vi "Rx Streaming Time (Host).vi"() -> ()   [LabVIEW 2021]
doc: "This template is for the Simple NI-USRP Streaming design, a design that shows the basics of streaming data to and from an NI USRP-294x/295x device. Refer to the block diagram for more information about how to use this template."
uses:
  Host/SubVIs/Start Trigger.ctl
  <extravilib>/ChannelInstances/Tag-c(bool,i32,str).lvlib
  <extravilib>/ChannelInstances/Stream-u32.lvlib
  <extravilib>/ChannelInstances/Tag-bool.lvlib
  <vilib>/userDefined/Silver/nirio_resource_slv.ctl
panel:
  out "acquiring":bool caption="Streaming"
  out "write time":u32[](graph)
  in  "max queue size":i32=100
  out "record time (ms)":u32
  out "write rate (SPS)":dbl format="%#_6p"
  out "# elements in queue":i32
  out "write tdms loop time (ms)":u32
  in  "frequency":dbl=2000000000.0 format="%#_6p"
  in  "sample rate":i32=50000000 format="%.0p"
  in  "start trigger":T1=enum."Immediate"
  out "get data loop time (ms)":u32 format="%.0p"
  out "error tdms_loop":errorcluster
  in  "USRP RIO device":T2="RIO0" caption="USRP RIO Device"
  in  "rx.stop":bool
  # "Overview: Demonstrates the use of the Advanced TDMS and simple streamer functions to write Rx data to a *.tdms file.\nInstructions:\nThis Vi must use Administrator privliges in order to write the data.\nthe USRP sohld be connected via MIXe to the computer (or other direct connection)\nset the params \nRun this VI.\ndue to the way the memory work after some time it can occer that the saveing rate will decrise."
  # "Rx Streaming"
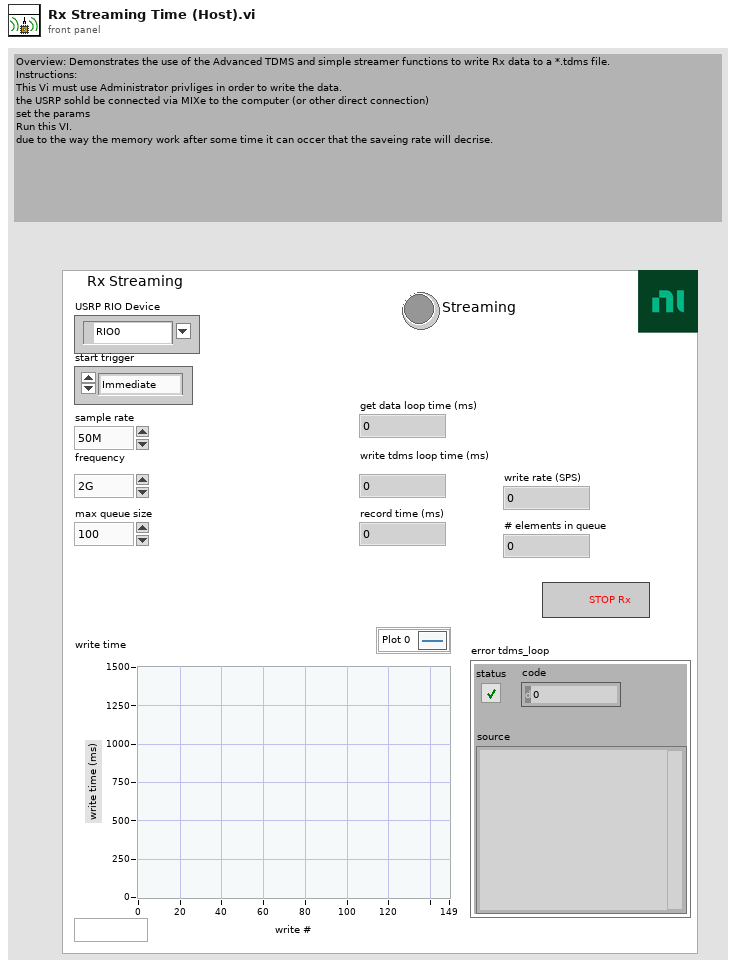
[diagram p1: front panel]
types:
  T1 = typedef "Start Trigger.ctl" = enum8{"Software", "Digital Edge", "Rx Start Trigger", "Tx Start Trigger", "Immediate", "Future Time Event"}
  T2 = typedef "nirio_resource_slv.ctl" = tag
  T3 = cluster{"rf enable 0":bool, "rf config 0":cluster{"antenna":string, "frequency":dbl, "lo frequency":dbl, "level":dbl}, "rf enable 1":bool, "rf config 1":cluster{"antenna":string, "frequency":dbl, "lo frequency":dbl, "level":dbl}, "transfer mode":enum16{"Finite", "Continuous"}, "sample rate":dbl, "number of samples":u32, "start trigger":T1}
  T4 = enum16{"open", "open or create", "create or replace", "create", "open (read-only)"}
  T5 = typedef "Rx Channels.ctl" = cluster{"rx config":cluster{"channel configuration":cluster{"channel enable":bool, "channel configuration":cluster{"antenna":string, "frequency":dbl, "lo frequency":dbl, "level":dbl}}[], "transfer mode":enum16{"Finite", "Continuous"}, "sample rate":dbl, "number of samples":u32, "start trigger":T1}, "reference frequency source":string, "rx.data sink":enum16{"SFP Port 0", "SFP Port 1", "Host"}, "rx.enabled channels":string[], "vertical range":dbl[], "rx.coerced configurations":cluster{"coerced frequencies":dbl[], "coerced lo frequencies":dbl[], "coerced levels":dbl[], "coerced sample rates":dbl[]}}
  T6 = typedef "niUsrpRio Config v1 Host.lvlib/niUsrpRio Session.ctl" = cluster{"FPGA Interface":refnum<k20>, "RIO Interface Number":u32, "Data Clock Rate":u32, "FPGA Data Clock Rate":u32, "Global Settings Register Bus":T7, "Radio 0 Settings Register Bus":T7, "Radio 1 Settings Register Bus":T7, "Radio Settings Bus Semaphore":T8, "DB Queues":T9[], "Characterization Data Valid?":bool, "EEPROM Header":T10, "Device Data Header":T11, "EEPROM Characterization Header":T12, "Characterization Data":T13[], "FPGA Current Version":u32, "FPGA Oldest Compatible Version":u32, "Fixed Logic Current Version":u32, "Fixed Logic Oldest Compatible Version":u32, "FPGA Radio Settings Bus Current Version":u32, "FPGA Radio Settings Bus Oldest Compatible Version":u32, "FPGA Board Config Current Version":u32, "FPGA Board Config Oldest Compatible Version":u32, "Daughterboard Clock Rate":u32, "daughterboard configuration session handles":u64[]}
  T7 = typedef "niInstr Register Bus v0 Host.lvlib/Register Bus Session.ctl" = refnum<queue>
  T8 = typedef "Semaphore RefNum" = refnum<k1>
  T9 = typedef "niUsrpRio Config v1 Host.lvlib/DB Queue Reference.ctl" = refnum<queue>
  T10 = typedef "niUsrpRio Config v1 Host.lvlib/EEPROM Header.ctl" = cluster{"Checksum":u32, "Product Code":u16, "Hardware Current Version":u16, "Hardware Oldest Compatible Version":u16, "EEPROM Map Current Version":u16, "EEPROM Map Oldest Compatible Version":u16, "User Password":string, "Pointer to Factory Header":u32, "Pointer to User Header":u32, "Recommended Interval":u16, "Number of Reserved Bytes":i32, "Number of Daughterboards":u8, "Daughterboard IDs":u16[], "Daughterboard Serial Numbers":string[]}
  T11 = typedef "niUsrpRio Config v1 Host.lvlib/EEPROM Device Data Header.ctl" = cluster{"Checksum":u32, "Number of Channels":u8, "Number of Gain Settings":u16[], "Pointer to Characterization Data":u32[], "Number of Reserved Bytes":i32, "Number of Frequencies":u16[]}
  T12 = typedef "niUsrpRio Config v1 Host.lvlib/EEPROM Characterization Header.ctl" = cluster{"Checksum":u32, "Date":timestamp, "Temperature":sgl, "Misc. Info":string, "Pointer to Device Data Header":u32, "Number of Reserved Bytes":i32}
  T13 = typedef "niUsrpRio Config v1 Host.lvlib/Characterization Data.ctl" = cluster{"Gains[dB]":dbl[], "Frequencies [Hz]":dbl[], "IQ Imbalance Table":T14[], "Measured Gains[dB]":dbl[][]}
  T14 = typedef "niUsrpRio Config v1 Host.lvlib/IQ Imbalance.ctl" = cluster{"Gain Imbalance [linear]":dbl, "Phase Imbalance [radians]":dbl, "Offset":cdb}
  T15 = typedef "Tag-bool.lvlib/))Channel.ctl" = refnum<queue>
  T16 = typedef "Stream-u32.lvlib/)Channel.ctl" = refnum<queue>
  T17 = typedef "Tag-c(bool,i32,str).lvlib/))Channel.ctl" = refnum<queue>
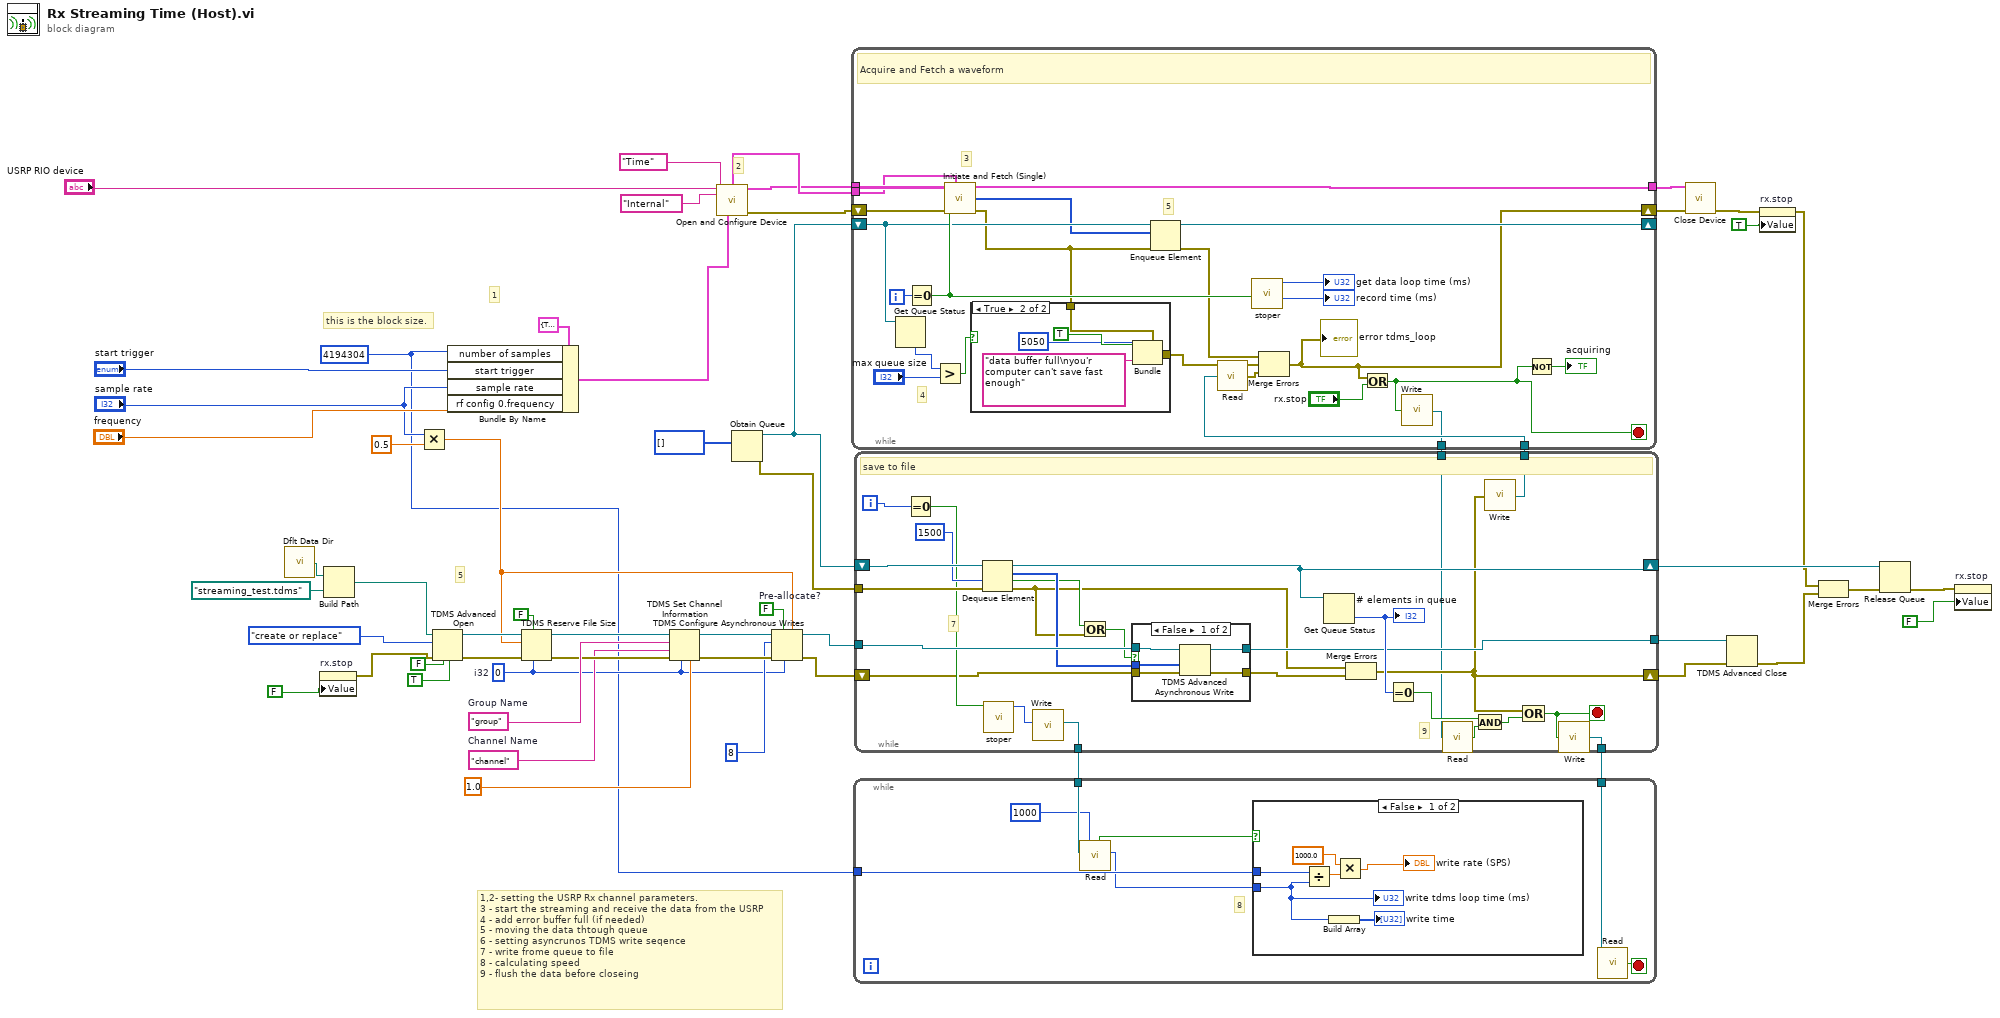
[diagram p0: block diagram]
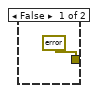
[diagram p3: hidden frame]
diagram:
  w5 = 4194304
  w43 = FALSE  # Pre-allocate?
  w21 = 0  # i32
  w54 = "group"  # Group Name
  w23 = "channel"  # Channel Name
  # "1,2- setting the USRP Rx channel parameters.\n3 - start the streaming and receive the data from the USRP\n4 - add error buffer full (if needed)\n5 - moving the data thtough queue   \n6 - setting asyncrunos TDMS write seqence\n7 - write frome queue to file\n8 - calculating speed\n9 - flush the data before closeing"
  # "5"
  # "2"
  # "1"
  # "this is the block size."
  n1 = call <vilib>:"Dflt Data Dir.vi"() -> ("App:Default Data Directory"=w10:path)
  n2 = property on="rx.stop" class="Bool (strict)"("Value"=FALSE) -> (error out=w16:errorcluster)  [unwired: 2 in, 1 out]
  n3 = Build Path(base path=w10, name or relative path=path "streaming_test.tdms") -> (appended path=w9:path)
  n4 = Multiply(x="sample rate", y=0.5) -> (x*y=w24:dbl)
  n5 = TDMS Advanced Open(4:TRUE ("enable asynchronous? (T)"), 6:FALSE ("disable buffering? (T)"), 8:w16, 10:T4."create or replace" ("operation (0:open)"), 11:w9) -> (0:w50:errorcluster, 3:w51:refnum<k34>)  [unwired: 1 out]
  n6 = Bundle By Name(cluster=T3 {"rf enable 0"=TRUE, "rf config 0"={"antenna"="RX1", "frequency"=2000000000.0, "lo frequency"=-1.0, "level"=0.0}, "rf enable 1"=FALSE, "rf config 1"={"antenna"="RX2", "frequency"=2000000000.0, "lo frequency"=-1.0, "level"=0.0}, "transfer mode"=enum."Continuous", "sample rate"=10000000.0, "number of samples"=4194304, "start trigger"=enum."Immediate"} ("rx config"), "number of samples"=w5, "start trigger"="start trigger", "sample rate"="sample rate", "rf config 0.frequency"="frequency") -> (w46:T3)
  n7 = TDMS Reserve File Size(6:w21, 7:FALSE ("append? (T)"), 8:w50, 10:w24, 11:w51) -> (0:w48:errorcluster, 3:w49:refnum<k34>)
  n8 = TDMS Set Channel Information(4:1.0 ("y"), 6:w21, 8:w48, 9:w23, 10:w54, 11:w49) -> (0:w45:errorcluster, 3:w44:refnum<k34>)  [unwired: 1 in]
  n9 = call "Open and Configure Device.vi"("USRP RIO Device"="USRP RIO device", "reference frequency source"="Internal", "which bitfile"="Time", "rx config"=w46) -> ("rx channels"=w56:T5, "niUsrpRio Session (out)"=w42:T6, "error out"=w41:errorcluster)  [unwired: 5 in, 4 out]
  n10 = Obtain Queue(element data type=u32[] [] ("waveform data")) -> (queue out=w30:refnum<queue>, error out=w29:errorcluster)  [unwired: 4 in, 1 out]
  n11 = TDMS Configure Asynchronous Writes(5:w24, 6:w21, 7:w43, 8:w45, 10:u32 8 ("max asynchronous writes (4)"), 11:w44) -> (0:w25:errorcluster, 3:w31:refnum<k34>)  [unwired: 1 in]
  n12 = while {
    tunnel: w42 -> [w78]
    tunnel: [w75] -> w32
    tunnel: w56 -> [w76]
    shift-right: [w74] -> _
    shift-left: w30 -> [w71]
    tunnel: w6 -> [w61]
    tunnel: [w60] -> w1
    shift-right: [w57] -> w8
    shift-left: w41 -> [w79]
    i -> [w80]
    stop <- w59 stop-if-true
    # "5"
    # "4"
    # "3"
    # "Acquire and Fetch a waveform"
    n13 = Get Queue Status(queue=w71) -> (# elements in queue=w70:i32)  [unwired: 2 in, 7 out]
    n14 = Equal To 0?(x=w80) -> (x = 0?=w77:bool)
    n15 = Greater?(x=w70, y="max queue size") -> (0:w68:bool)
    n16 = call "Initiate and Fetch (Single).vi"("niUsrpRio Session"=w78, "rx channels"=w76, "first iteration"=w77, "error in"=w79) -> ("niUsrpRio Session (out)"=w75:T6, "array w/ subset deleted"=w64:u32[], "error out"=w69:errorcluster)  [unwired: 9 in]
    n17 = case shown="True" w68 {
      tunnel: w69 -> [_ w86]
      tunnel: [errorcluster {"status"=FALSE, "code"=0, "source"=""} ("error out") w85] -> w67
      frame False {
      }
      frame True {
        n18 = Bundle(cluster=w86, "status"=TRUE, "code"=5050, "source"="data buffer full\nyou'r computer can't save fast enough") -> (w85:errorcluster)
      }
    }
    n19 = Enqueue Element(queue=w71, element=w64, error in (no error)=w69) -> (queue out=w74:refnum<queue>, error out=w72:errorcluster)  [unwired: 1 in, 1 out]
    n20 = call <extravilib>:"Read.vi"("channel"=w61) -> ("element"=w62:errorcluster)  [unwired: 1 in, 1 out]
    n21 = call "stoper.vi"("x mission"=w77) -> ("frome start"=→"record time (ms)":u32, "loop"=→"get data loop time (ms)":u32)  [unwired: 8 in, 1 out]
    n22 = Merge Errors(w72, w67, w62) -> (w57:errorcluster)
    "error tdms_loop" <- w57
    n23 = Or(x=w57, y="rx.stop") -> (x .or. y?=w59:bool)
    n24 = call <extravilib>:"Write.vi"("element"=w59) -> ("channel"=w60:T15)  [unwired: 1 out]
    n25 = Not(x=w59) -> (.not. x?=→"acquiring":bool)
  }
  n26 = while {
    tunnel: w31 -> [w104]
    shift-right: [w108] -> w26
    shift-left: w30 -> [w111]
    tunnel: w29 -> [w109]
    tunnel: [w102] -> w27
    shift-right: [w96] -> w14
    shift-left: w25 -> [w97]
    tunnel: [w95] -> w6
    tunnel: [w93] -> w4
    tunnel: [w92] -> w3
    tunnel: w1 -> [w88]
    i -> [w99]
    stop <- w110 stop-if-true
    # "9"
    # "7"
    # "save to file"
    n27 = Equal To 0?(x=w99) -> (x = 0?=w98:bool)
    n28 = Dequeue Element(queue=w111, timeout in ms (-1)=1500, error in (no error)=w109) -> (queue out=w108:refnum<queue>, element=w101:u32[], timed out?=w91:bool, error out=w90:errorcluster)
    n29 = call "stoper.vi"("x mission"=w98) -> ("loop"=w94:u32)  [unwired: 8 in, 2 out]
    n30 = call <extravilib>:"Write.vi"("element"=w94) -> ("channel"=w93:T16)  [unwired: 8 in, 2 out]
    n31 = Or(x=w91, y=w90) -> (x .or. y?=w89:bool)
    n32 = case shown="False" w89 {
      tunnel: w104 -> [w116 w118]
      tunnel: [w115 w117] -> w103
      tunnel: [w114 w118] -> w102
      tunnel: w101 -> [w113 _]
      tunnel: w97 -> [w112 w117]
      frame False {
        n33 = TDMS Advanced Asynchronous Write(8:w112, 10:w113, 11:w116) -> (0:w115:errorcluster, 3:w114:refnum<k34>)
      }
      frame True {
      }
    }
    n34 = Get Queue Status(queue=w108) -> (# elements in queue=w107:i32)  [unwired: 2 in, 7 out]
    "# elements in queue" <- w107
    n35 = Merge Errors(w90, w103) -> (w96:errorcluster)
    n36 = Equal To 0?(x=w107) -> (x = 0?=w106:bool)
    n37 = call <extravilib>:"Read.vi"("channel"=w88) -> ("element"=w87:bool)  [unwired: 1 in, 1 out]
    n38 = And(x=w106, y=w87) -> (x .and. y?=w105:bool)
    n39 = call <extravilib>:"Write.vi"("element"=w96) -> ("channel"=w95:T17)  [unwired: 1 out]
    n40 = Compound Arithmetic op=OR(w96, w105) -> (w110:bool)
    n41 = call <extravilib>:"Write.vi"("element"=w110) -> ("channel"=w92:T15)  [unwired: 1 out]
  }
  n42 = while {
    tunnel: w5 -> [w125]
    tunnel: w4 -> [w124]
    tunnel: w3 -> [w120]
    stop <- w119 stop-if-true
    # "8"
    n43 = call <extravilib>:"Read.vi"("timeout in ms (-1)"=1000, "channel"=w124) -> ("element"=w123:u32, "timed out?"=w121:bool)  [unwired: 5 in, 3 out]
    n44 = case shown="False" w121 {
      tunnel: w125 -> [w131 _]
      tunnel: w123 -> [w130 _]
      frame False {
        n45 = Divide(x=w131, y=w130) -> (x/y=w127:dbl)
        n46 = Build Array(w130) -> (→"write time":u32[])
        n47 = Multiply(x=1000.0, y=w127) -> (x*y=→"write rate (SPS)":dbl)
        "write tdms loop time (ms)" <- w130
      }
      frame True {
      }
    }
    n48 = call <extravilib>:"Read.vi"("channel"=w120) -> ("element"=w119:bool)  [unwired: 1 in, 1 out]
  }
  n49 = call "Close Device.vi"("niUsrpRio Session"=w32, "error in"=w8) -> ("error out"=w15:errorcluster)  [unwired: 13 in]
  n50 = TDMS Advanced Close(8:w14, 11:w27) -> (0:w13:errorcluster)  [unwired: 2 in, 1 out]
  n51 = property on="rx.stop" class="Bool (strict)"(error in=w15, "Value"=TRUE) -> (error out=w7:errorcluster)  [unwired: 1 in, 1 out]
  n52 = Merge Errors(w7, w13) -> (w17:errorcluster)
  n53 = Release Queue(queue=w26, error in (no error)=w17) -> (error out=w2:errorcluster)  [unwired: 1 in, 2 out]
  n54 = property on="rx.stop" class="Bool (strict)"(error in=w2, "Value"=FALSE) -> ()  [unwired: 1 in, 2 out]
